vi "LUT.vi"(11 "Hub Distance (ft)":dbl) -> (2 "Hood Setpoint":dbl, 3 "Shooter RPM":dbl)   [LabVIEW 2025]
panel:
  out "Fractional Index":dbl
  out "Step Size":i32
  out "Start Distance":i32
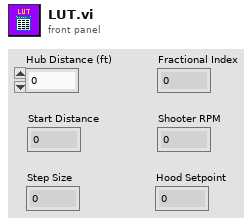
[diagram p1: front panel]
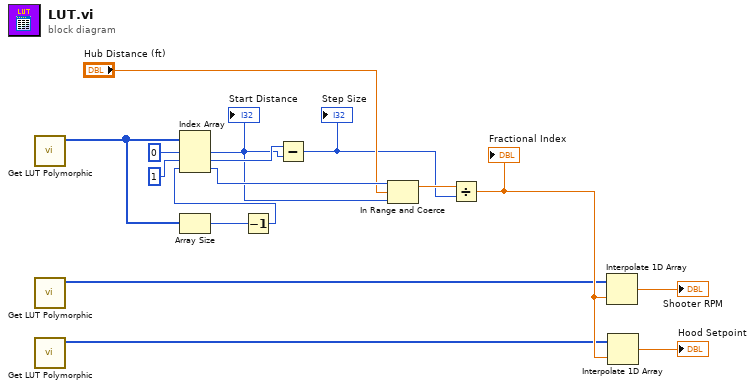
[diagram p0: block diagram]
diagram:
  n1 = call-poly "Get LUT Polymorphic.vi"() -> ("LUT Out"=w3:i32[])  [unwired: 10 in, 1 out]
  n2 = call-poly "Get LUT Polymorphic.vi"() -> ("LUT Out"=w2:i32[])  [unwired: 10 in, 1 out]
  n3 = call-poly "Get LUT Polymorphic.vi"() -> ("LUT Out"=w1:i32[])  [unwired: 10 in, 1 out]
  n4 = Array Size(array=w3) -> (size(s)=w13:i32)
  n5 = Decrement(x=w13) -> (x-1=w12:i32)
  n6 = Index Array(array=w3, index #1=0 ("index"), index #2=1 ("index"), index #3=w12) -> (element #1=w10:i32, element #2=w14:i32, element #3=w11:i32)
  "Start Distance" <- w10
  n7 = Subtract(x=w14, y=w10) -> (x-y=w7:i32)
  "Step Size" <- w7
  n8 = In Range and Coerce(upper limit=w11, x="Hub Distance (ft)", lower limit=w10) -> (coerced(x)=w8:dbl)  [unwired: 1 out]
  n9 = Divide(x=w8, y=w7) -> (x/y=w5:dbl)
  "Fractional Index" <- w5
  n10 = Interpolate 1D Array(1:w5, 2:w2) -> (0:→"Shooter RPM":dbl)
  n11 = Interpolate 1D Array(1:w5, 2:w1) -> (0:→"Hood Setpoint":dbl)
